vi "Derivative of XY graph.vi"() -> ()   [LabVIEW 2016]
uses:
  <vilib>/Analysis/NI_AALPro.lvlib
panel:
  out "Data number":i32=4304
  out "Decay time vs G [ (G/(dG/dt)) vs G ]":cluster{dbl[], dbl[]}[](graph)
  out "Portion of curve":cluster{dbl[], dbl[]}[](graph)
  in  "Cluster":T1={"start index"=41262, "end index"=45565, "Plot portion of curve?"=TRUE}
  in  "Name":T2={"X"="Time (s)", "Y"="2-T G (S)", "dY/dX"="Decay Slope (S/s)", "dX/dY"="N/A"}
  out "array size":i32=62598
  out "Derivative graph":cluster{dbl[], dbl[]}[](graph)
  in  "Y axis":enum16{"dY/dX", "dX/dY"}(ring)
  in  "X axis":enum16{"Y", "X"}(ring)
  in  "Step for derivative":dbl=102.0
  in  "2T-G":cluster{dbl[], dbl[]}[](graph)=[{array[62598 elements], array[62598 elements]}]
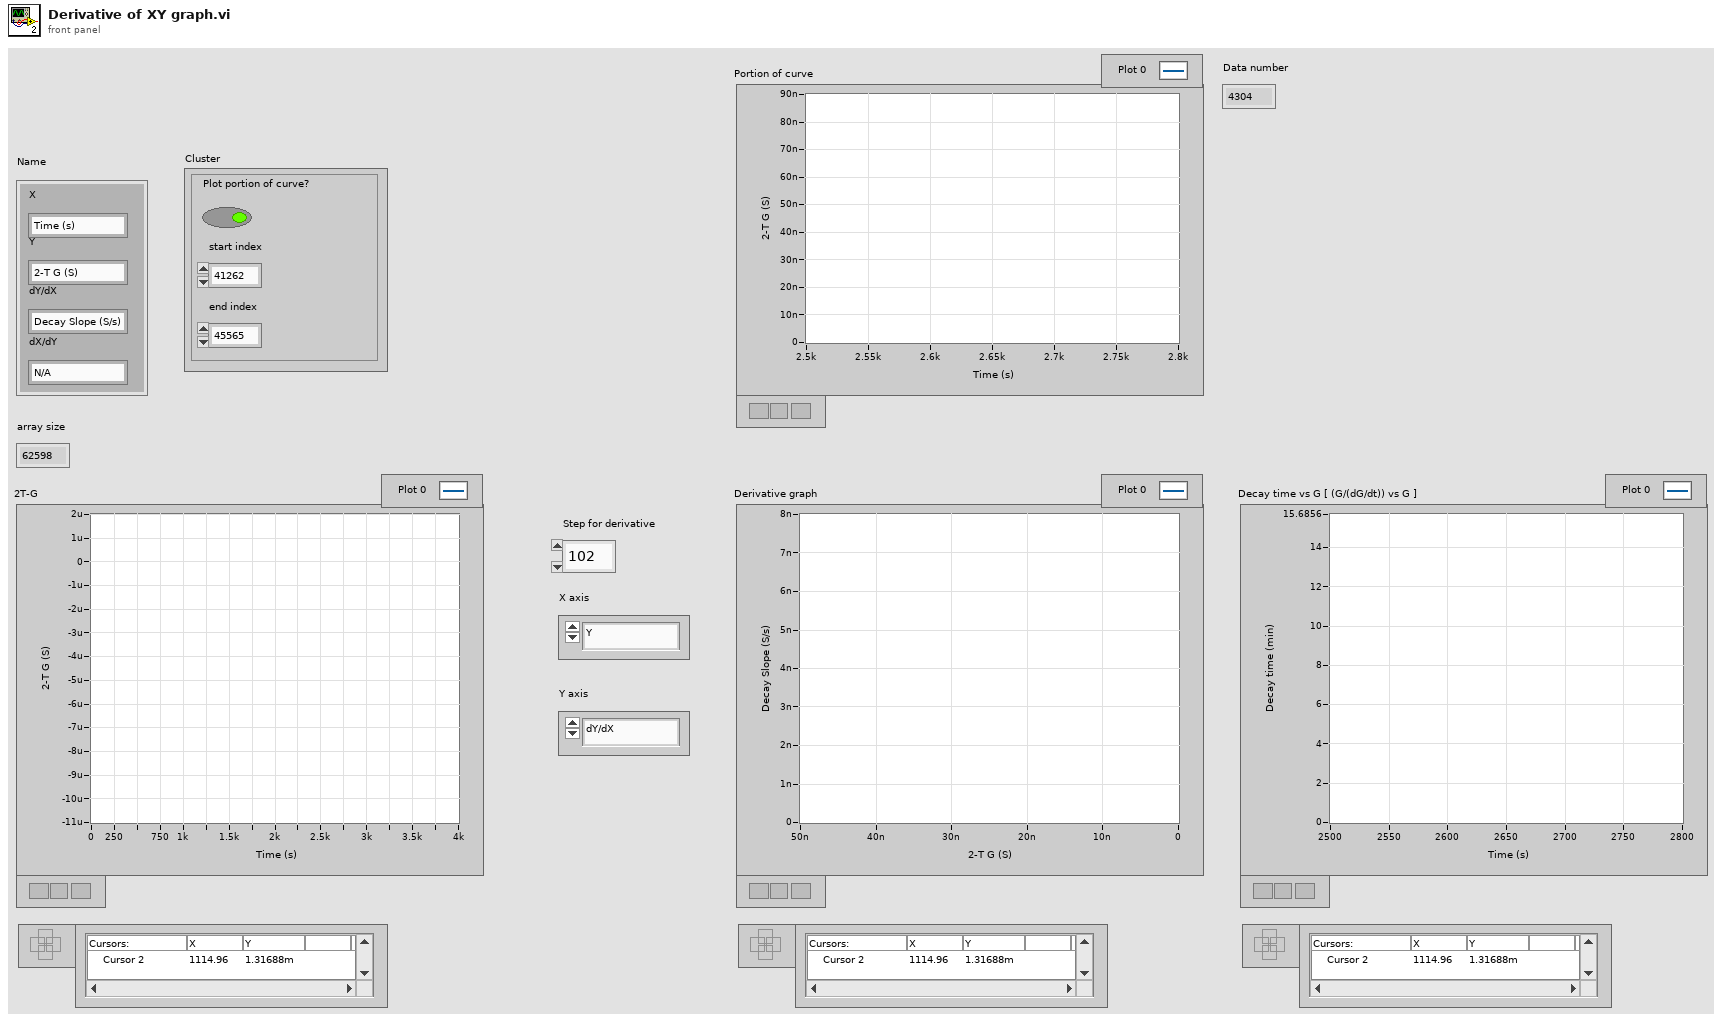
[diagram p1: front panel]
types:
  T1 = cluster{"start index":i32, "end index":i32, "Plot portion of curve?":bool}
  T2 = cluster{"X":string, "Y":string, "dY/dX":string, "dX/dY":string}
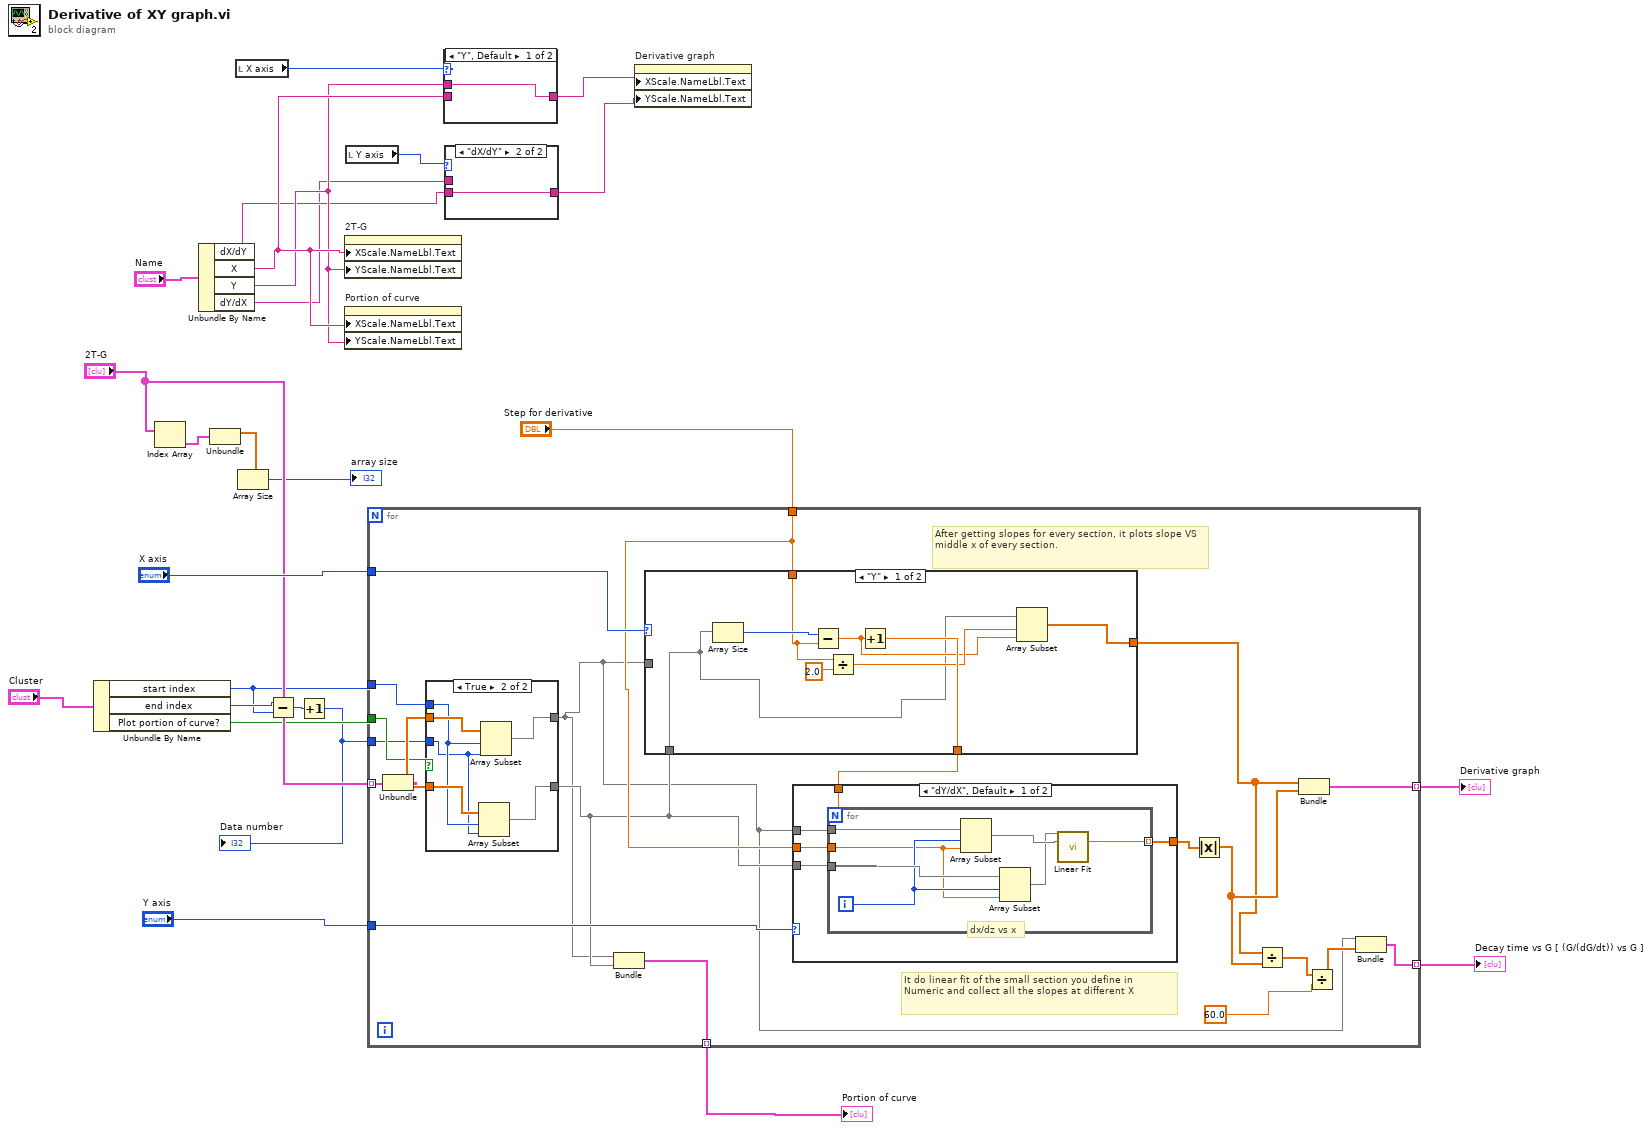
[diagram p0: block diagram]
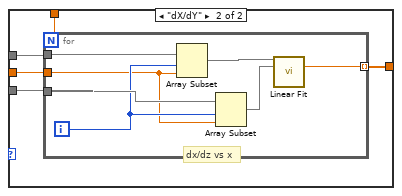
[diagram p5: hidden frame]
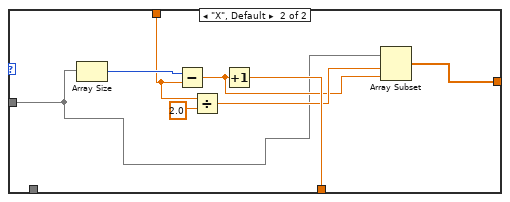
[diagram p6: hidden frame]
diagram:
  n1 = Unbundle By Name("Cluster") -> ("start index"=w14:i32, "end index"=w15:i32, "Plot portion of curve?"=w16:bool)
  n2 = Index Array(array="2T-G") -> (element=w20:cluster{dbl[], dbl[]})  [unwired: 1 in]
  n3 = Unbundle By Name("Name") -> ("dX/dY"=w4:string, "X"=w8:string, "Y"=w5:string, "dY/dX"=w2:string)
  n4 = Unbundle(w20) -> (w19:dbl[])  [unwired: 1 out]
  n5 = local read "X axis"() -> (w9:enum16{"Y", "X"})
  n6 = Array Size(array=w19) -> (size(s)=→"array size":i32)
  n7 = Subtract(x=w15, y=w14) -> (x-y=w13:i32)
  n8 = Increment(x=w13) -> (x+1=w12:i32)
  "Data number" <- w12
  n9 = property on="2T-G" class="XYGraph (strict)"("XScale.NameLbl.Text"=w8, "YScale.NameLbl.Text"=w5) -> ()  [unwired: 2 in, 2 out]
  n10 = property on="Portion of curve" class="XYGraph (strict)"("XScale.NameLbl.Text"=w8, "YScale.NameLbl.Text"=w5) -> ()  [unwired: 2 in, 2 out]
  n11 = local read "Y axis"() -> (w6:enum16{"dY/dX", "dX/dY"})
  n12 = for {
    tunnel: [w46] -> w22 mode=indexing
    tunnel: "2T-G" -> [w41] mode=indexing
    tunnel: "Step for derivative" -> [w42]
    tunnel: "X axis" -> [w45]
    tunnel: "Y axis" -> [w43]
    tunnel: w16 -> [w38]
    tunnel: w14 -> [w37]
    tunnel: w12 -> [w36]
    tunnel: [w34] -> w11 mode=indexing
    tunnel: [w30] -> w1 mode=indexing
    # "After getting slopes for every section, it plots slope VS middle x of every section."
    # "It do linear fit of the small section you define in Numeric and collect all the slopes at different X"
    n13 = Unbundle(w41) -> (w40:dbl[], w39:dbl[])
    n14 = case shown="True" w38 {
      tunnel: w40 -> [w48 w54]
      tunnel: [w48 w53] -> w26
      tunnel: w39 -> [w47 w52]
      tunnel: [w47 w51] -> w35
      tunnel: w37 -> [_ w50]
      tunnel: w36 -> [_ w49]
      frame False {
      }
      frame True {
        n15 = Array Subset(array=w52, index=w50, length=w49) -> (w51:dbl[])
        n16 = Array Subset(array=w54, index=w50, length=w49) -> (w53:dbl[])
      }
    }
    n17 = Bundle(w26, w35) -> (w34:cluster{dbl[], dbl[]})  [unwired: 1 in]
    n18 = case shown="\"Y\"" w45 {
      tunnel: [w86 w94] -> w44
      tunnel: [w80 w88] -> w27
      tunnel: w26 -> [_ w87]
      tunnel: w42 -> [w81 w89]
      tunnel: w35 -> [w79 _]
      frame "Y" {
        n19 = Array Size(array=w79) -> (size(s)=w82:i32)
        n20 = Subtract(x=w82, y=w81) -> (x-y=w83:dbl)
        n21 = Divide(x=w81, y=2.0) -> (x/y=w84:dbl)
        n22 = Increment(x=w83) -> (x+1=w86:dbl)
        n23 = Array Subset(array=w79, index=w84, length=w83) -> (w80:dbl[])
      }
      frame "X", Default {
        n24 = Array Size(array=w87) -> (size(s)=w90:i32)
        n25 = Subtract(x=w90, y=w89) -> (x-y=w91:dbl)
        n26 = Divide(x=w89, y=2.0) -> (x/y=w92:dbl)
        n27 = Increment(x=w91) -> (x+1=w94:dbl)
        n28 = Array Subset(array=w87, index=w92, length=w91) -> (w88:dbl[])
      }
    }
    n29 = case shown="\"dY/dX\", Default" w43 {
      tunnel: [w59 w71] -> w33
      tunnel: w26 -> [w58 w70]
      tunnel: w35 -> [w57 w69]
      tunnel: w42 -> [w56 w68]
      tunnel: w44 -> [w55 w67]
      frame "dY/dX", Default {
        # "dx/dz vs x"
        n30 = for {
          N: w55 -> [_]
          tunnel: w58 -> [w66]
          tunnel: w57 -> [w65]
          tunnel: w56 -> [w63]
          tunnel: [w62] -> w59 mode=indexing
          i -> [w64]
          n31 = Array Subset(array=w66, index=w64, length=w63) -> (w61:dbl[])
          n32 = Array Subset(array=w65, index=w64, length=w63) -> (w60:dbl[])
          n33 = call <vilib>:"Linear Fit.vi"("Y"=w60, "X"=w61) -> ("slope"=w62:dbl)  [unwired: 9 in, 4 out]
        }
      }
      frame "dX/dY" {
        # "dx/dz vs x"
        n34 = for {
          N: w67 -> [_]
          tunnel: w70 -> [w78]
          tunnel: w69 -> [w77]
          tunnel: w68 -> [w75]
          tunnel: [w74] -> w71 mode=indexing
          i -> [w76]
          n35 = Array Subset(array=w78, index=w76, length=w75) -> (w73:dbl[])
          n36 = Array Subset(array=w77, index=w76, length=w75) -> (w72:dbl[])
          n37 = call <vilib>:"Linear Fit.vi"("Y"=w73, "X"=w72) -> ("slope"=w74:dbl)  [unwired: 9 in, 4 out]
        }
      }
    }
    n38 = Absolute Value(x=w33) -> (abs(x)=w32:dbl[])
    n39 = Divide(x=w27, y=w32) -> (x/y=w31:dbl[])
    n40 = Bundle(w27, w32) -> (w46:cluster{dbl[], dbl[]})  [unwired: 1 in]
    n41 = Divide(x=w31, y=60.0) -> (x/y=w29:dbl[])
    n42 = Bundle(w26, w29) -> (w30:cluster{dbl[], dbl[]})  [unwired: 1 in]
  }
  "Derivative graph" <- w22
  "Portion of curve" <- w11
  "Decay time vs G [ (G/(dG/dt)) vs G ]" <- w1
  n43 = case shown="\"Y\", Default" w9 {
    tunnel: w8 -> [_ w96]
    tunnel: [w95 w96] -> w7
    tunnel: w5 -> [w95 _]
    frame "Y", Default {
    }
    frame "X" {
    }
  }
  n44 = case shown="\"dX/dY\"" w6 {
    tunnel: w4 -> [_ w98]
    tunnel: [w97 w98] -> w3
    tunnel: w2 -> [w97 _]
    frame "dY/dX", Default {
    }
    frame "dX/dY" {
    }
  }
  n45 = property on="Derivative graph" class="XYGraph (strict)"("XScale.NameLbl.Text"=w7, "YScale.NameLbl.Text"=w3) -> ()  [unwired: 2 in, 2 out]
